vi "SetParam.vi"(8 "error in (no error)":errorcluster caption="entrée d'erreur (pas d'erreur)", 10 "PolynomialFeatures":T1={"degre"=2, "interaction_only"=FALSE, "include_bias"=TRUE, "order"="C"}, 11 "PolynomialFeatures.lvclass":refnum<class "PolynomialFeatures.lvclass">) -> (0 "error out":errorcluster caption="sortie d'erreur", 3 "PolynomialFeatures.lvclass":refnum<class "PolynomialFeatures.lvclass">)   [LabVIEW 2020, in "PolynomialFeatures.lvclass"]
doc: "Set Parameters"
uses:
  PolynomialFeatures.lvclass
  PolynomialFeatures.lvclass/PolynomialFeatures.ctl
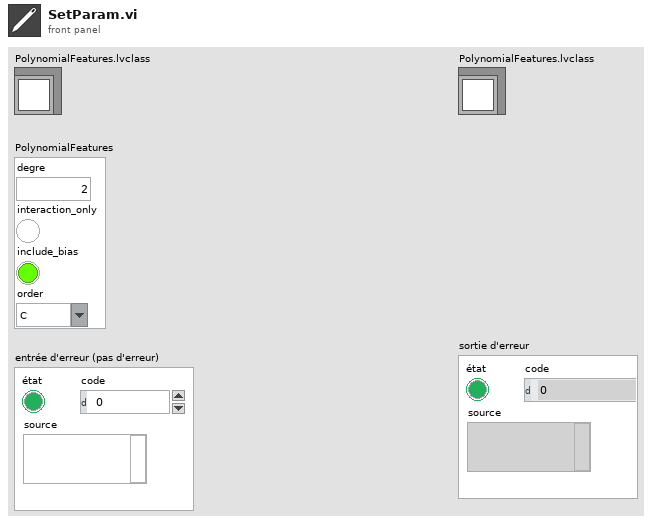
[diagram p1: front panel]
types:
  T1 = cluster{"degre":i32, "interaction_only":bool, "include_bias":bool, "order":string}
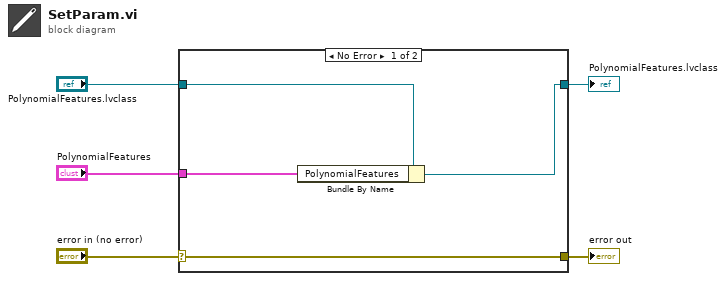
[diagram p0: block diagram]
diagram:
  n1 = case shown="No Error" "error in (no error)" {
    selector: "error in (no error)" -> [w9 w10]
    tunnel: [w9 w10] -> w4
    tunnel: [w7 w11] -> w2
    tunnel: "PolynomialFeatures.lvclass" -> [w8 w11]
    tunnel: "PolynomialFeatures" -> [w6 _]
    frame No Error {
      n2 = Bundle By Name(cluster=w8, "PolynomialFeatures"=w6) -> (w7:refnum<class "PolynomialFeatures.lvclass">)
    }
    frame Error {
    }
  }
  "error out" <- w4
  "PolynomialFeatures.lvclass" <- w2
